vi "Window-Dialogue-Set origin.vi"(7 "Colour":u32(colorbox)=16777225, 8 "error in (no error)":errorcluster, 9 "Caption-Left button (Cancel)":string, 10 "Caption-Right button (OK)":string, 11 "Message string":string) -> (0 "error out":errorcluster, 1 "Cancelled (Left button pressed)":bool)   [LabVIEW 2013]
doc: "Use this template to create a dialog box with event handling."
uses:
  <vilib>/Utility/miscctls.llb/LVPointTypeDef.ctl
  Global Variables/General Globals.vi
panel:
  in  "Left Button":bool
  in  "Rigth Button":bool
  out "Message":string
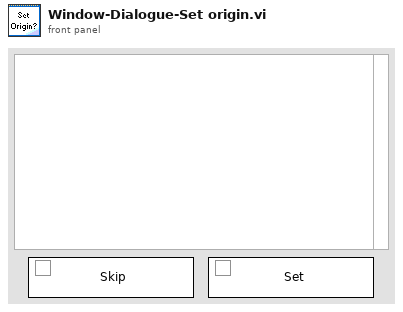
[diagram p1: front panel]
types:
  T1 = typedef "LVPointTypeDef.ctl" = cluster{"Horizontal":i16, "Vertical":i16}
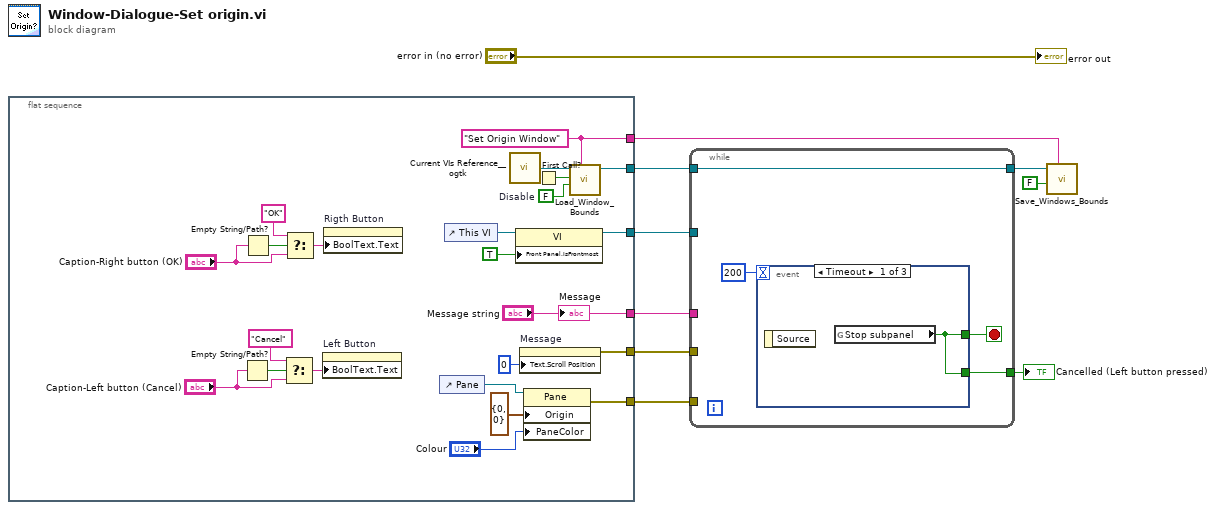
[diagram p0: block diagram]
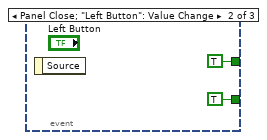
[diagram p2: hidden frame]
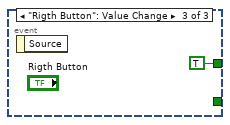
[diagram p3: hidden frame]
diagram:
  n1 = flat-sequence {
    tunnel: ["Message string"] -> w10
    tunnel: [w31] -> w9
    tunnel: [w28] -> w8
    tunnel: [w26] -> w7
    tunnel: [w21] -> w5
    tunnel: [w20] -> w3
    frame #0 {
      w22 = FALSE  # Disable
      w21 = "Set Origin Window" ("Window Name (i.e. Key)")
      n2 = Empty String/Path?(string/path="Caption-Left button (Cancel)") -> (empty?=w14:bool)
      n3 = Empty String/Path?(string/path="Caption-Right button (OK)") -> (empty?=w18:bool)
      n4 = Select(t="Cancel", s=w14, f="Caption-Left button (Cancel)") -> (s? t:f=w13:string)
      n5 = Select(t="OK", s=w18, f="Caption-Right button (OK)") -> (s? t:f=w16:string)
      n6 = property on="Left Button" class="Bool"("BoolText.Text"=w13) -> ()  [unwired: 2 in, 2 out]
      n7 = property on="Rigth Button" class="Bool"("BoolText.Text"=w16) -> ()  [unwired: 2 in, 2 out]
      n8 = control-ref of="Pane"() -> (w25:refnum<vi>)
      n9 = control-ref of="This VI"() -> (w29:refnum<vi>)
      n10 = call "Current VIs Reference__ogtk.vi"() -> ("Current VI's reference"=w24:refnum<vi>)  [unwired: 5 in]
      n11 = property on="Property Node" class="VI"(reference=w29, "Front Panel.IsFrontmost"=TRUE ("Front Panel Window:Is Frontmost")) -> (reference out=w28:refnum<vi>)  [unwired: 1 in, 1 out]
      n12 = property on="Message" class="Str"("Text.Scroll Position"=u32 0) -> (error out=w31:errorcluster)  [unwired: 2 in, 1 out]
      n13 = property class="Pane"(reference=w25, "Origin"=T1 {"Horizontal"=0, "Vertical"=0}, "PaneColor"="Colour") -> (error out=w26:errorcluster)  [unwired: 1 in, 1 out]
      n14 = First Call?() -> (First Call?: T/F=w23:bool)
      n15 = call "Load_Window_Bounds.vi"("Window Name (i.e. Key)"=w21, "Disable"=w22, "First Call"=w23, "Window VI's Ref"=w24) -> ("reference out"=w20:refnum<vi>)  [unwired: 4 in, 3 out]
      "Message" <- "Message string"
    }
  }
  n16 = while {
    tunnel: w10 -> [_]
    tunnel: w9 -> [_]
    tunnel: w7 -> [_]
    tunnel: w8 -> [_]
    tunnel: [w35] -> w6
    tunnel: w3 -> [w34]
    tunnel: [w34] -> w2
    stop <- w37 stop-if-true
    n17 = event shown="[0] Timeout" {
      selector: _ -> [_ _ _]
      dyn-events: _ -> [_ _ _]
      timeout: 200 -> [_ _ _]
      tunnel: [w38 TRUE ("Stop?") TRUE ("Stop?")] -> w37
      tunnel: [w38 TRUE ("Stop subpanel") _] -> w35
      event Timeout {
        n18 = event-data() -> ()  [unwired: 1 in, 1 out]
        n19 = global read "General Globals.vi" "Stop subpanel"() -> (w38:bool)
      }
      event Panel Close; "Left Button": Value Change {
        n20 = event-data() -> ()  [unwired: 1 in, 1 out]
      }
      event "Rigth Button": Value Change {
        n21 = event-data() -> ()  [unwired: 1 in, 1 out]
      }
    }
  }
  "Cancelled (Left button pressed)" <- w6
  n22 = call "Save_Windows_Bounds.vi"("Window Name (i.e. Key)"=w5, "Front Panel Window:Open"=FALSE, "Window VI's Ref"=w2) -> ()  [unwired: 8 in, 1 out]
  "error out" <- "error in (no error)"
